vi "Call_test.vi"   [LabVIEW 2015]
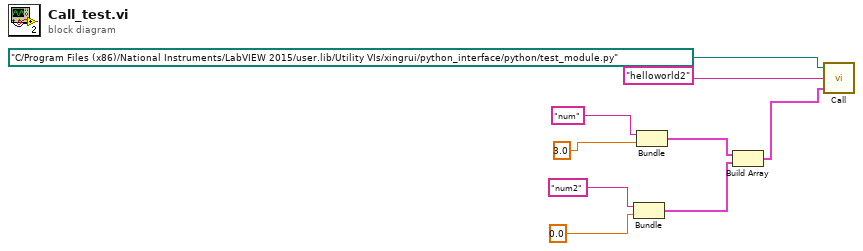
[diagram p0: block diagram]
diagram:
  n1 = Bundle("num2", 0.0) -> (w4:cluster{string, dbl})  [unwired: 1 in]
  n2 = Bundle("num", 3.0) -> (w5:cluster{string, dbl})  [unwired: 1 in]
  n3 = Build Array(w5, w4) -> (w1:cluster{string, dbl}[])
  n4 = call <userlib>:"Call.vi"("Arguments"=w1, "Function or Method Name"="helloworld2", "Path to Python Module (.py file)"=path "C:/Program Files (x86)/National Instruments/LabVIEW 2015/user.lib/Utility VIs/xingrui/python_interface/python/test_module.py") -> ()
